vi "Override.vi"(2 "Invert":bool, 9 "Regualer":dbl, 11 "Override":bool, 13 "Overriden":dbl) -> (15 "Output":dbl)   [LabVIEW 2012]
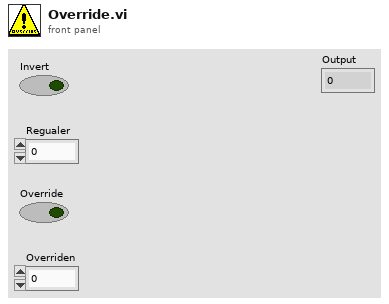
[diagram p1: front panel]
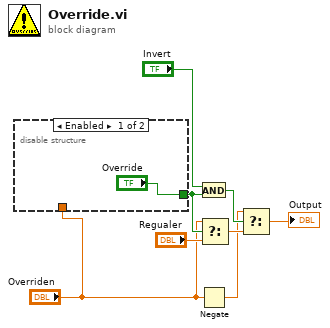
[diagram p0: block diagram]
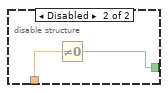
[diagram p2: hidden frame]
diagram:
  n1 = disable-structure shown="Enabled" {
    disable-tunnel: ["Override" w10] -> w6
    disable-tunnel: "Overriden" -> [_ w11]
    frame Enabled {
    }
    frame Disabled {
      n2 = Not Equal To 0?(x=w11) -> (x != 0?=w10:bool)
    }
  }
  n3 = And(x="Invert", y=w6) -> (x .and. y?=w4:bool)
  n4 = Negate(x="Overriden") -> (-x=w3:dbl)
  n5 = Select(t="Overriden", s=w6, f="Regualer") -> (s? t:f=w8:dbl)
  n6 = Select(t=w3, s=w4, f=w8) -> (s? t:f=→"Output":dbl)
